vi "Render.vi"(8 "error in (no error)":errorcluster, 10 "String in":string, 11 "Line in":refnum<class "Line.lvclass">) -> (0 "error out":errorcluster, 2 "String out":string, 3 "Line out":refnum<class "Line.lvclass">)   [LabVIEW 2021, in "Markdown.lvlib" / "Line.lvclass"]
uses:
  Line.lvclass
  C:/GitHub/Markdown/src/Markdown/Markdown.lvclass
  Line.lvclass/Line.ctl
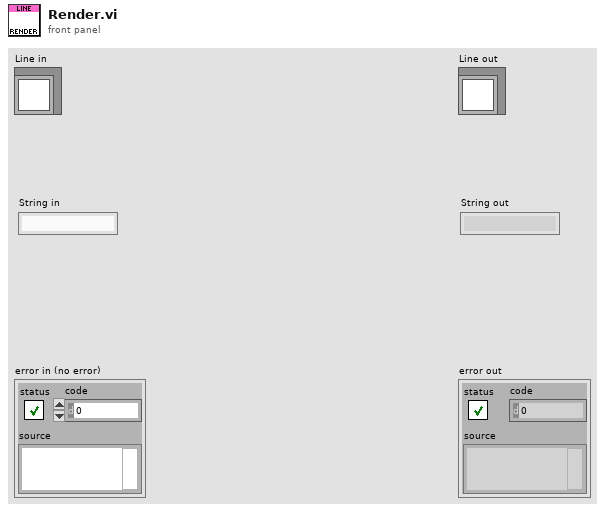
[diagram p1: front panel]
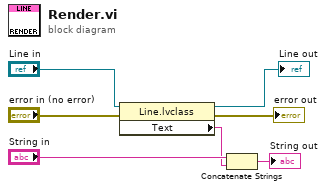
[diagram p0: block diagram]
diagram:
  n1 = property class="Line.lvclass"(reference="Line in", error in="error in (no error)") -> (reference out=→"Line out":refnum<class "Line.lvclass">, error out=→"error out":errorcluster, "Text"=w4:string)
  n2 = Concatenate Strings("String in", w4) -> (→"String out":string)
